vi "ymode分包.vi"(1 "文件（使用对话框）":path) -> (0 "分包数组":string[](array[string]))   [LabVIEW 2015]
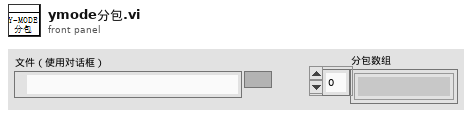
[diagram p1: front panel]
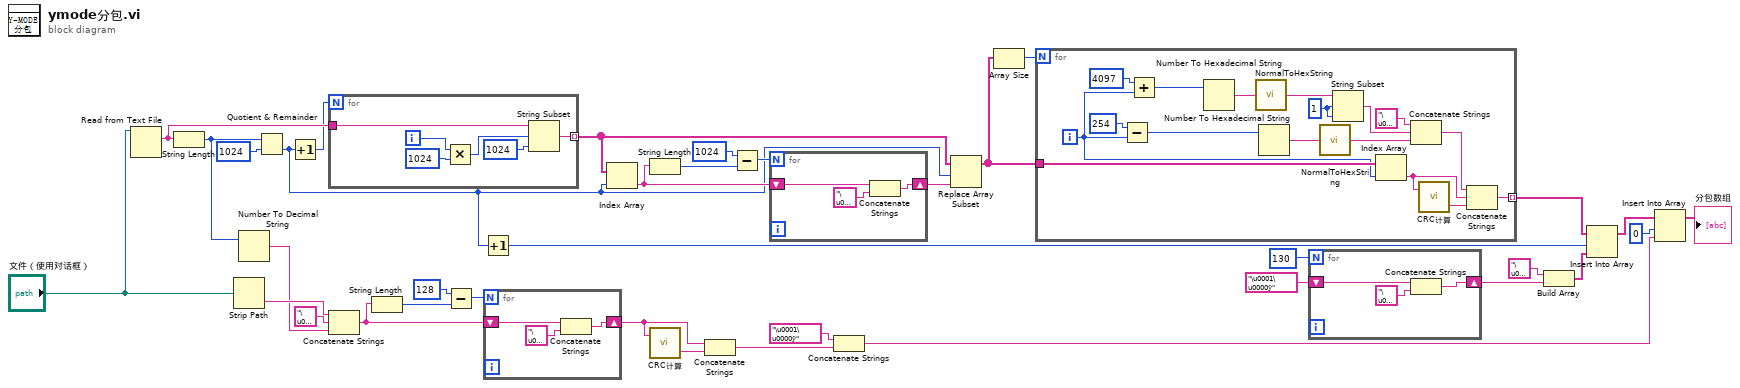
[diagram p0: block diagram]
diagram:
  n1 = Read from Text File(file (use dialog)="文件（使用对话框）") -> (text=w35:string)  [unwired: 3 in, 3 out]
  n2 = String Length(string=w35) -> (length=w5:i32)
  n3 = Strip Path(path="文件（使用对话框）") -> (name=w24:string)  [unwired: 1 out]
  n4 = Number To Decimal String(number=w5) -> (decimal integer string=w22:string)  [unwired: 1 in]
  n5 = Quotient & Remainder(x=w5, y=1024) -> (floor(x/y)=w10:i32)  [unwired: 1 out]
  n6 = Increment(x=w10) -> (x+1=w28:i32)
  n7 = for {
    N: w28 -> [_]
    tunnel: w35 -> [w42]
    tunnel: [w38] -> w29 mode=indexing
    i -> [w37]
    n8 = Multiply(x=w37, y=1024) -> (x*y=w40:i32)
    n9 = String Subset(string=w42, offset (0)=w40, length (rest)=1024) -> (substring=w38:string)
  }
  n10 = Concatenate Strings(w24, "\u0000", w22) -> (w18:string)
  n11 = String Length(string=w18) -> (length=w20:i32)
  n12 = Subtract(x=128, y=w20) -> (x-y=w19:i32)
  n13 = Increment(x=w10) -> (x+1=w9:i32)
  n14 = for {
    N: w19 -> [_]
    shift-right: [w43] -> w17
    shift-left: w18 -> [w45]
    n15 = Concatenate Strings(w45, "\u0000") -> (w43:string)
  }
  n16 = Index Array(array=w29, index=w10) -> (element=w31:string)
  n17 = String Length(string=w31) -> (length=w34:i32)
  n18 = call "CRC计算.vi"("需要检验的字符串（以16进制显示的字符串）"=w17) -> ("CRC校验位"=w16:string)  [unwired: 1 in, 1 out]
  n19 = Concatenate Strings(w17, w16) -> (w14:string)
  n20 = Subtract(x=1024, y=w34) -> (x-y=w32:i32)
  n21 = for {
    N: w32 -> [_]
    shift-right: [w46] -> w30
    shift-left: w31 -> [w48]
    n22 = Concatenate Strings(w48, "\u001a") -> (w46:string)
  }
  n23 = Concatenate Strings("\u0001\u0000ÿ", w14) -> (w12:string)
  n24 = Replace Array Subset(array=w29, new element=w30, index=w10) -> (w26:string[])
  n25 = Array Size(array=w26) -> (size(s)=w27:i32)
  n26 = for {
    N: w27 -> [_]
    tunnel: w26 -> [w54]
    tunnel: [w50] -> w11 mode=indexing
    i -> [w53]
    w63 = 1
    n27 = Subtract(x=254, y=w53) -> (x-y=w57:i32)
    n28 = Add(x=4097, y=w53) -> (x+y=w56:i32)
    n29 = Number To Hexadecimal String(2:w56) -> (0:w62:string)  [unwired: 1 in]
    n30 = call "NormalToHexString.vi"("Normal Display String"=w62) -> ("Hex Display String"=w65:string)  [unwired: 14 in]
    n31 = Number To Hexadecimal String(2:w57) -> (0:w58:string)  [unwired: 1 in]
    n32 = call "NormalToHexString.vi"("Normal Display String"=w58) -> ("Hex Display String"=w60:string)  [unwired: 14 in]
    n33 = String Subset(string=w65, offset (0)=w63, length (rest)=w63) -> (substring=w64:string)
    n34 = Index Array(array=w54, index=w53) -> (element=w52:string)
    n35 = Concatenate Strings("\u0002", w64, w60) -> (w51:string)
    n36 = call "CRC计算.vi"("需要检验的字符串（以16进制显示的字符串）"=w52) -> ("CRC校验位"=w49:string)  [unwired: 1 in, 1 out]
    n37 = Concatenate Strings(w51, w52, w49) -> (w50:string)
  }
  n38 = for {
    N: 130 -> [_]
    shift-right: [w66] -> w2
    shift-left: "\u0001\u0000ÿ" -> [w68]
    n39 = Concatenate Strings(w68, "\u0000") -> (w66:string)
  }
  n40 = Build Array("\u0004", w2) -> (w7:string[])
  n41 = Insert Into Array(array=w11, index=w9, new element=w7) -> (w6:string[])
  n42 = Insert Into Array(array=w6, index=0, new element=w12) -> (→"分包数组":string[])
